vi "3020仪器参数发送.vi"   [LabVIEW 2016, in "数据传输系统-06.lvlib"]
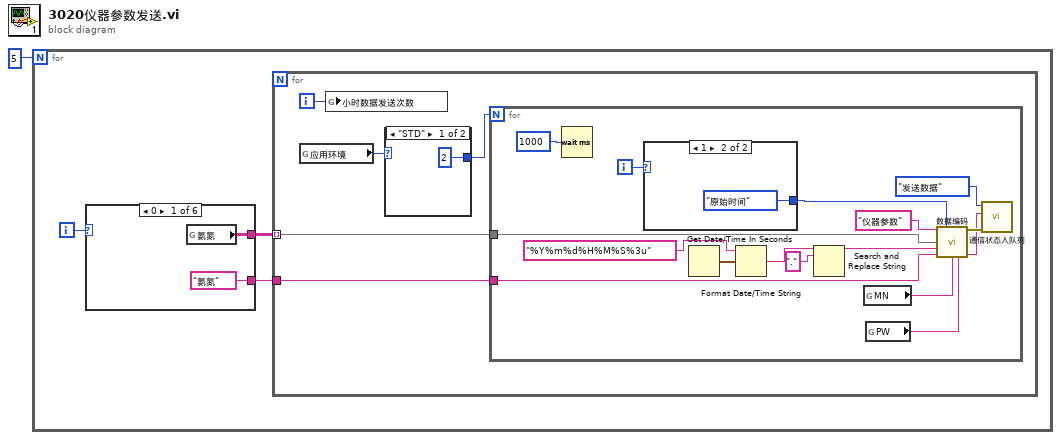
[diagram p0: block diagram]
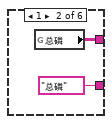
[diagram p2: hidden frame]
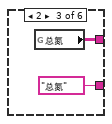
[diagram p3: hidden frame]
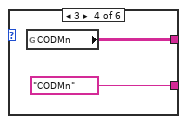
[diagram p4: hidden frame]
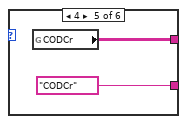
[diagram p5: hidden frame]
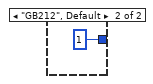
[diagram p7: hidden frame]
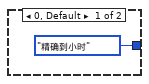
[diagram p8: hidden frame]
diagram:
  n1 = for {
    N: 5 -> [_]
    i -> [w4]
    n2 = case shown="0" w4 {
      tunnel: [w6 w8 w10 w12 w14 _] -> w3
      tunnel: ["氨氮" ("污染物编码") "总磷" ("污染物编码") "总氮" ("污染物编码") "CODMn" ("污染物编码") "CODCr" ("污染物编码") _] -> w2
      frame 0 {
        n3 = global read "全局 所有参数.vi" "氨氮"() -> (w6:string[][])
      }
      frame 1 {
        n4 = global read "全局 所有参数.vi" "总磷"() -> (w8:string[][])
      }
      frame 2 {
        n5 = global read "全局 所有参数.vi" "总氮"() -> (w10:string[][])
      }
      frame 3 {
        n6 = global read "全局 所有参数.vi" "CODMn"() -> (w12:string[][])
      }
      frame 4 {
        n7 = global read "全局 所有参数.vi" "CODCr"() -> (w14:string[][])
      }
      frame 5, Default {
      }
    }
    n8 = for {
      tunnel: w2 -> [w19]
      tunnel: w3 -> [w18] mode=indexing
      i -> [w17]
      n9 = global read "断电保存全局.vi" "应用环境"() -> (w15:enum16{"STD", "GB212"})
      n10 = global write "全局 小时数据发送次数.vi" "小时数据发送次数"(w17) -> ()
      n11 = case shown="\"STD\"" w15 {
        tunnel: [2 1] -> w16
        frame "STD" {
        }
        frame "GB212", Default {
        }
      }
      n12 = for {
        N: w16 -> [_]
        tunnel: w19 -> [w28]
        tunnel: w18 -> [w27]
        i -> [w25]
        n13 = Wait (ms)(milliseconds to wait=u32 1000 ("等待时间（毫秒）")) -> ()  [unwired: 1 out]
        n14 = case shown="1" w25 {
          tunnel: [enum16{"精确到小时", "原始时间"}."精确到小时" ("仪器参数上传时间") enum16{"精确到小时", "原始时间"}."原始时间" ("仪器参数上传时间")] -> w24
          frame 0, Default {
          }
          frame 1 {
          }
        }
        n15 = Get Date/Time In Seconds() -> (seconds since 1Jan1904=w35:timestamp)
        n16 = Format Date/Time String(time format string (%c)="%Y%m%d%H%M%S%3u" ("时间格式字符串(%c)"), seconds (now)=w35) -> (date/time string=w34:string)  [unwired: 1 in]
        n17 = Search and Replace String(input string=w34, search string="." ("搜索字符串")) -> (result string=w32:string)  [unwired: 6 in, 3 out]
        n18 = global read "断电保存全局.vi" "MN"() -> (w31:string)
        n19 = global read "断电保存全局.vi" "PW"() -> (w30:string)
        n20 = call "数据编码.vi"("table输入"="仪器参数" ("新元素/子数组"), "仪器参数上传时间"=w24, "仪器参数"=w27, "QN"=w32, "参数"=w28, "MN"=w31, "PW"=w30) -> ("错误常量"=w29:errorcluster, "通讯包字符串"=w22:string)  [unwired: 7 in]
        n21 = call "通信状态入队列.vi"("错误输入（无错误）"=w29, "发送报文"=w22, "枚举"=enum16{"打开连接", "发送数据", "读取数据", "数据处理", "关闭连接"}."发送数据") -> ()  [unwired: 8 in, 1 out]
      }
    }
  }
